vi "WT200 GET Harmonics.vi"(8 "error in (no error)":errorcluster, 11 "VISA Refnum in":refnum<visa-resource-name>) -> (0 "error out":errorcluster, 1 "VTHD":dbl, 2 "Final Harmonic Content U1":string, 3 "VISA Refnum out":refnum<visa-resource-name>)   [LabVIEW 2016]
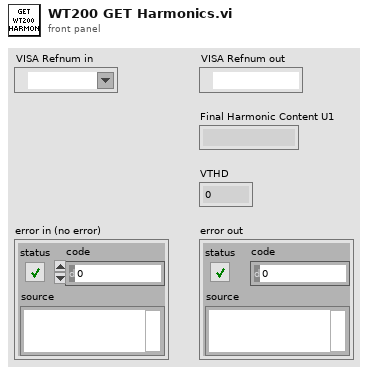
[diagram p1: front panel]
types:
  T1 = typedef "YOKOGAWA Options.ctl" = cluster{"GP-IB Communication /C1":bool, "Ethernet Communication /C7":bool, "External Current Sensor /EX1":bool, "External Current Sensor /EX2":bool, "External Current Sensor /EX3":bool, "VGA Output /V1":bool, "Harmonic Measurment /G5":bool, "Delta Computation /DT":bool, "Added Frequency Measurment /FQ":bool, "Serial Interface /C2":bool, "D/A Output /DA4":bool, "D/A Output /DA12":bool, "Comparator Output /CMP":bool}
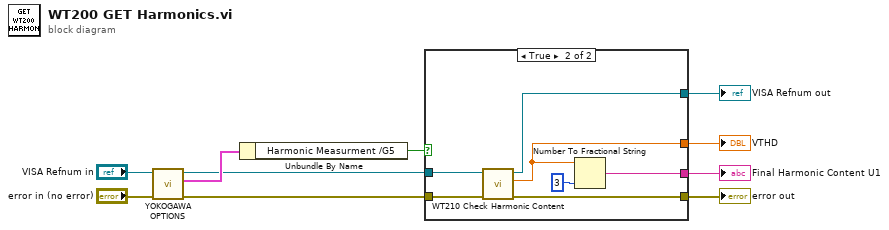
[diagram p0: block diagram]
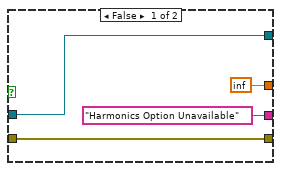
[diagram p2: hidden frame]
diagram:
  n1 = call "YOKOGAWA OPTIONS.vi"("Error In"="error in (no error)", "VISA resource name"="VISA Refnum in") -> ("Error Out"=w5:errorcluster, "Yokogawa Options"=w7:T1, "VISA resource name out"=w6:refnum<visa-resource-name>)  [unwired: 7 in]
  n2 = Unbundle By Name(w7) -> ("Harmonic Measurment /G5"=w9:bool)
  n3 = case shown="True" w9 {
    tunnel: [w13 w21] -> w1
    tunnel: [w14 w20] -> w2
    tunnel: w5 -> [w14 w19]
    tunnel: w6 -> [w13 w18]
    tunnel: [inf w16] -> w8
    tunnel: ["Harmonics Option Unavailable" w15] -> w10
    frame False {
    }
    frame True {
      n4 = call "WT210 Check Harmonic Content.vi"("error in (no error)"=w19, "VISA Refnum in"=w18) -> ("error out"=w20:errorcluster, "VTHD"=w16:sgl, "VISA Refnum out"=w21:refnum<visa-resource-name>)  [unwired: 7 in]
      n5 = Number To Fractional String(number=w16, precision (6)=i16 3) -> (F-format string=w15:string)  [unwired: 2 in]
    }
  }
  "Final Harmonic Content U1" <- w10
  "VTHD" <- w8
  "error out" <- w2
  "VISA Refnum out" <- w1
